vi "Go.vi"(9 "Timing Values":dbl[](array[numeric]), 10 "Control In":T1={"I-O.lvclass"=refnum, "Motion.lvclass"=refnum, "Dispenser.lvclass"=refnum}, 11 "CAD Dispense in":refnum<class "CAD Dispense.lvclass">) -> (2 "Control Out":T1, 3 "CAD Dispense Out":refnum<class "CAD Dispense.lvclass">)   [LabVIEW 2016, in "CAD Dispense.lvclass"]
uses:
  CAD Dispense.lvclass
  Controller/Controllers.ctl
  Controller/I-O/I-O.lvclass
  Controller/Motion/A3200/A3200.lvclass
  Controller/Dispenser/Dispenser.lvclass
  Controller/Motion/Motion.lvclass
  CAD Dispense.lvclass/CAD Dispense.ctl
  Controller/Controller.lvclass
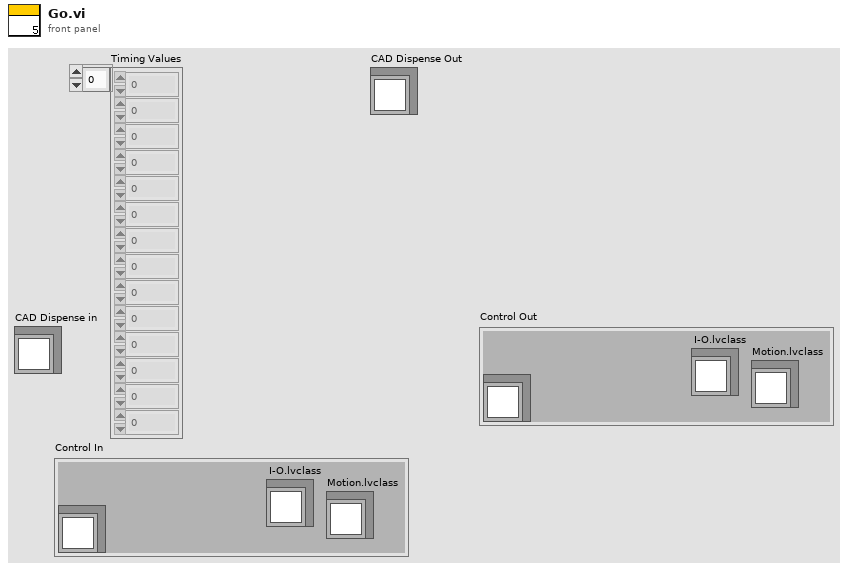
[diagram p1: front panel]
types:
  T1 = typedef "Controller.lvclass/Controllers.ctl" = cluster{"I-O.lvclass":refnum<class "I-O.lvclass">, "Motion.lvclass":refnum<class "Motion.lvclass">, "Dispenser.lvclass":refnum<class "Dispenser.lvclass">}
  T2 = cluster{"Motion":dbl[][], "Center":dbl[], "Circle?":bool, "CW/CCW":dbl}[]
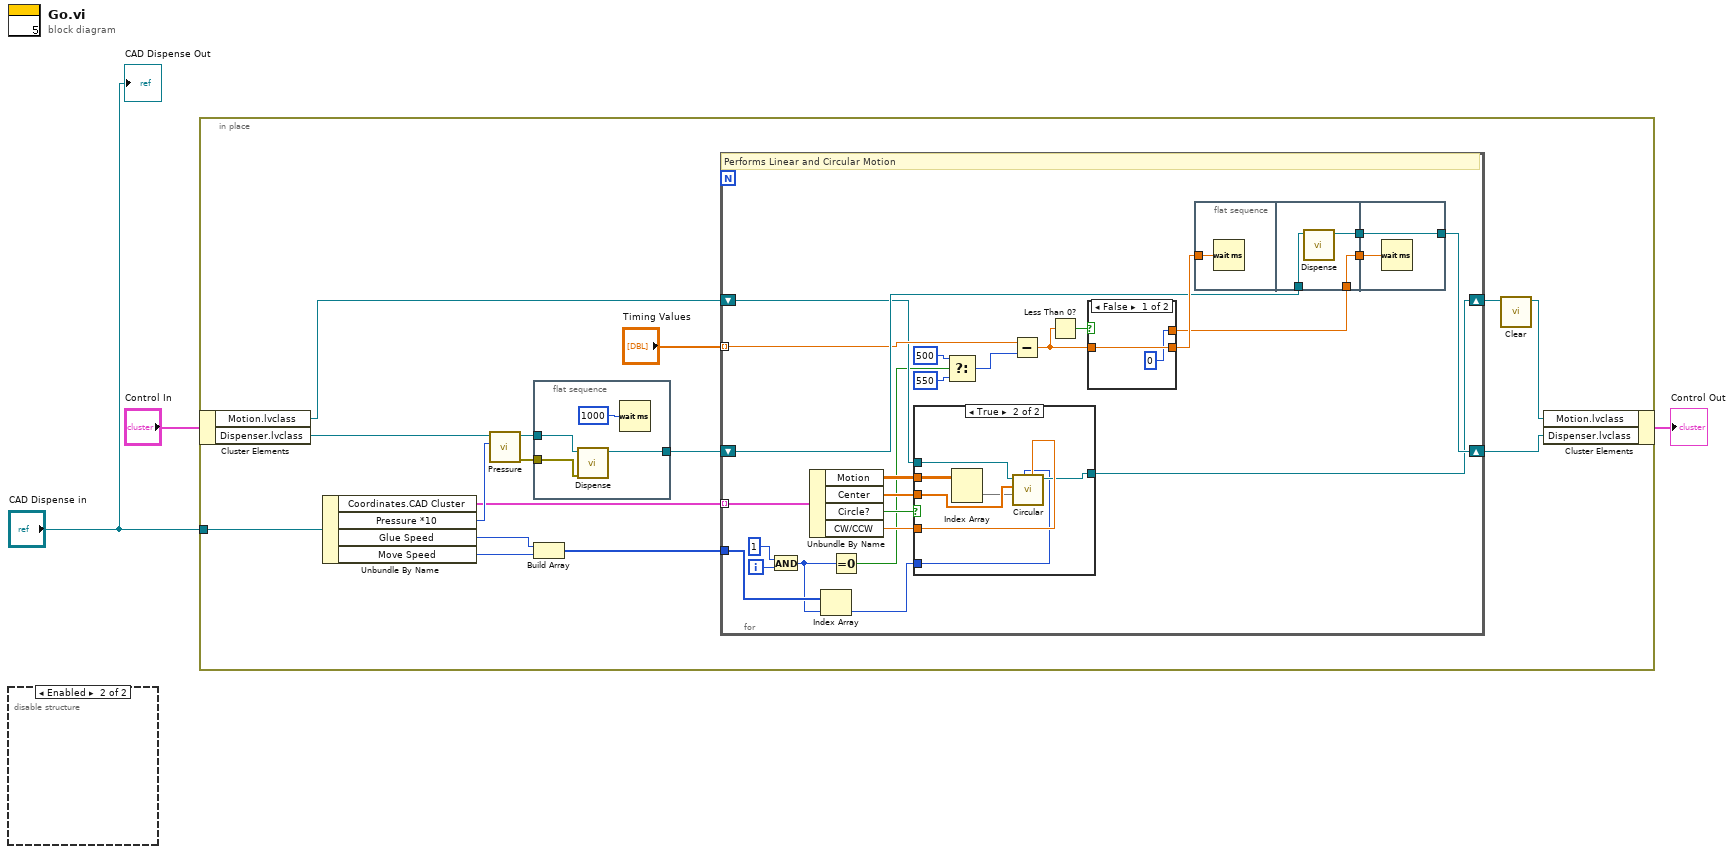
[diagram p0: block diagram]
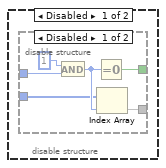
[diagram p2: hidden frame]
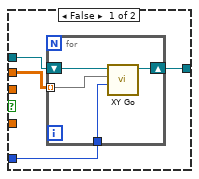
[diagram p4: hidden frame]
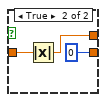
[diagram p5: hidden frame]
diagram:
  n1 = disable-structure shown="Enabled" {
    frame Disabled {
      n2 = disable-structure shown="Disabled" {
        disable-tunnel: [w8 _] -> _
        disable-tunnel: _ -> [w7 _]
        disable-tunnel: [w5 _] -> _
        disable-tunnel: _ -> [w4 _]
        frame Disabled {
          n3 = And(x=1, y=w7) -> (x .and. y?=w6:i32)
          n4 = Equal To 0?(x=w6) -> (x = 0?=w5:bool)
          n5 = Index Array(array=w4, index=w6) -> (element=w8)
        }
        frame Enabled {
        }
      }
    }
    frame Enabled {
    }
  }
  n6 = in-place {
    in-place-border: "CAD Dispense in" -> [w23]
    n7 = in-place-cluster #1("Control In") -> ("Motion.lvclass"=w17:refnum<class "Motion.lvclass">, "Dispenser.lvclass"=w14:refnum<class "Dispenser.lvclass">)
    n8 = Unbundle By Name(w23) -> ("Coordinates.CAD Cluster"=w10:T2, "Pressure *10"=w13:i64, "Glue Speed"=w21:i32, "Move Speed"=w20:i32)
    n9 = call-dynamic "Pressure.vi"("Pressure"=w13, "Dispenser in"=w14) -> ("error out"=w12:errorcluster, "Dispenser out"=w11:refnum<class "Dispenser.lvclass">)  [unwired: 8 in]
    n10 = flat-sequence {
      tunnel: [w26] -> w22
      tunnel: w12 -> [w25]
      tunnel: w11 -> [w27]
      frame #0 {
        n11 = call-dynamic "Dispense.vi"("error in (no error)"=w25, "Dispenser in"=w27) -> ("Dispenser out"=w26:refnum<class "Dispenser.lvclass">)  [unwired: 8 in, 1 out]
        n12 = Wait (ms)(milliseconds to wait=u32 1000) -> ()  [unwired: 1 out]
      }
    }
    n13 = Build Array(w21, w20) -> (w19:i32[])
    n14 = for {
      tunnel: w10 -> [w46] mode=indexing
      tunnel: "Timing Values" -> [w42] mode=indexing
      tunnel: w19 -> [w36]
      shift-right: [w39] -> w24
      shift-left: w22 -> [w48]
      shift-right: [w38] -> w16
      shift-left: w17 -> [w41]
      i -> [w35]
      # "Performs Linear and Circular Motion"
      n15 = And(x=1, y=w35) -> (x .and. y?=w33:i32)
      n16 = Unbundle By Name(w46) -> ("Motion"=w45:dbl[][], "Center"=w44:dbl[], "Circle?"=w37:bool, "CW/CCW"=w40:dbl)
      n17 = Index Array(array=w36, index=w33) -> (element=w29:i32)
      n18 = Equal To 0?(x=w33) -> (x = 0?=w32:bool)
      n19 = case shown="True" w37 {
        tunnel: [w57 w63] -> w38
        tunnel: w40 -> [_ w65]
        tunnel: w45 -> [w55 w68]
        tunnel: w44 -> [_ w67]
        tunnel: w41 -> [w56 w64]
        tunnel: w29 -> [w54 w62]
        frame False {
          n20 = for {
            tunnel: w55 -> [w59] mode=indexing
            shift-right: [w60] -> w57
            shift-left: w56 -> [w61]
            tunnel: w54 -> [w58]
            n21 = call-dynamic "XY Go.vi"("Speed"=w58, "XY"=w59, "Motion in"=w61) -> ("Motion out"=w60:refnum<class "Motion.lvclass">)  [unwired: 7 in, 1 out]
          }
        }
        frame True {
          n22 = Index Array(array=w68) -> (element=w66:dbl[])  [unwired: 2 in]
          n23 = call-dynamic "Circular.vi"("Direction"=w65, "Speed"=w62, "XY End"=w66, "XY Center"=w67, "Motion in"=w64) -> ("Motion out"=w63:refnum<class "Motion.lvclass">)  [unwired: 5 in, 1 out]
        }
      }
      n24 = Select(t=500, s=w32, f=550) -> (s? t:f=w47:i32)
      n25 = Subtract(x=w42, y=w47) -> (x-y=w43:dbl)
      n26 = Less Than 0?(x=w43) -> (x < 0?=w53:bool)
      n27 = case shown="False" w53 {
        tunnel: [w76 u32 0 ("milliseconds to wait")] -> w52
        tunnel: w43 -> [w76 w79]
        tunnel: [u32 0 ("milliseconds to wait") w78] -> w51
        frame False {
        }
        frame True {
          n28 = Absolute Value(x=w79) -> (abs(x)=w78:dbl)
        }
      }
      n29 = flat-sequence {
        tunnel: w52 -> [w69]
        tunnel: w48 -> [w71]
        tunnel: [w72] -> w50
        tunnel: w51 -> [w72]
        tunnel: [w70] -> w49
        tunnel: w50 -> [w74]
        tunnel: w49 -> [w73]
        tunnel: [w73] -> w39
        frame #0 {
          n30 = Wait (ms)(milliseconds to wait=w69) -> ()  [unwired: 1 out]
        }
        frame #1 {
          n31 = call-dynamic "Dispense.vi"("Dispenser in"=w71) -> ("Dispenser out"=w70:refnum<class "Dispenser.lvclass">)  [unwired: 9 in, 1 out]
        }
        frame #2 {
          n32 = Wait (ms)(milliseconds to wait=w74) -> ()  [unwired: 1 out]
        }
      }
    }
    n33 = call "Clear.vi"("Motion in"=w16) -> ("Motion out"=w15:refnum<class "Motion.lvclass">)  [unwired: 9 in, 1 out]
    n34 = in-place-cluster #1("Motion.lvclass"=w15, "Dispenser.lvclass"=w24) -> (→"Control Out":T1)
  }
  "CAD Dispense Out" <- "CAD Dispense in"
